vi "counter_control_multitap.vi"(0 "Downtime for pulse active":u32=20, 1 "Duration Pulse active":u32=10, 2 "Signal-high duration":u32=20, 3 "Signal-high lead-up":u32=10) -> ()   [LabVIEW 2015]
panel:
  out "Num Pulse errors":T1
  out "Configuration Error messages":T1
  # "Output"
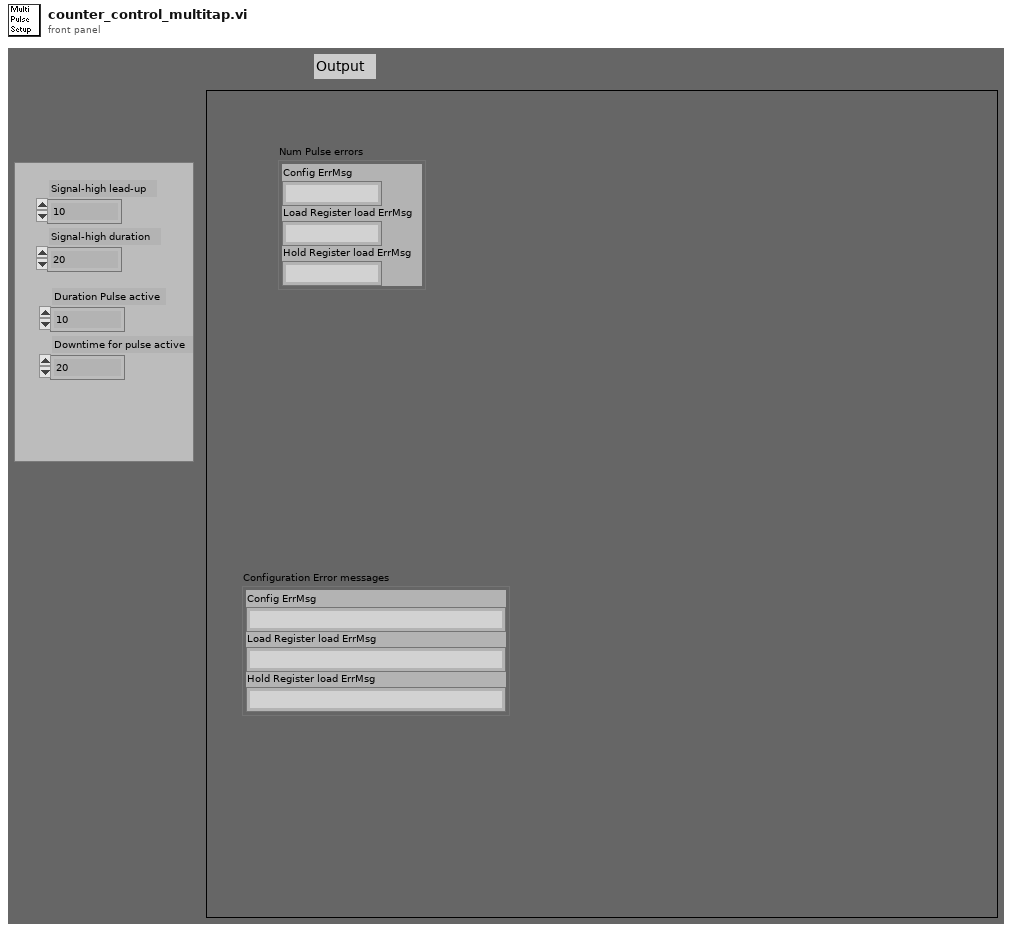
[diagram p1: front panel]
types:
  T1 = cluster{"Config ErrMsg":string, "Load Register load ErrMsg":string, "Hold Register load ErrMsg":string}
  T2 = cluster{"CounterNum":u32, "GateControl":u32, "CountSource Freq":u32, "OutputControl (LOW)":u32, "Signal-high lead-up":u32, "Signal-high duration":u32}
  T3 = cluster{"CounterNum":u32, "GateControl":u32, "CountSource Freq":u32, "OutputControl (LOW)":u32, "Duration Pulse active":u32, "Downtime for pulse active":u32}
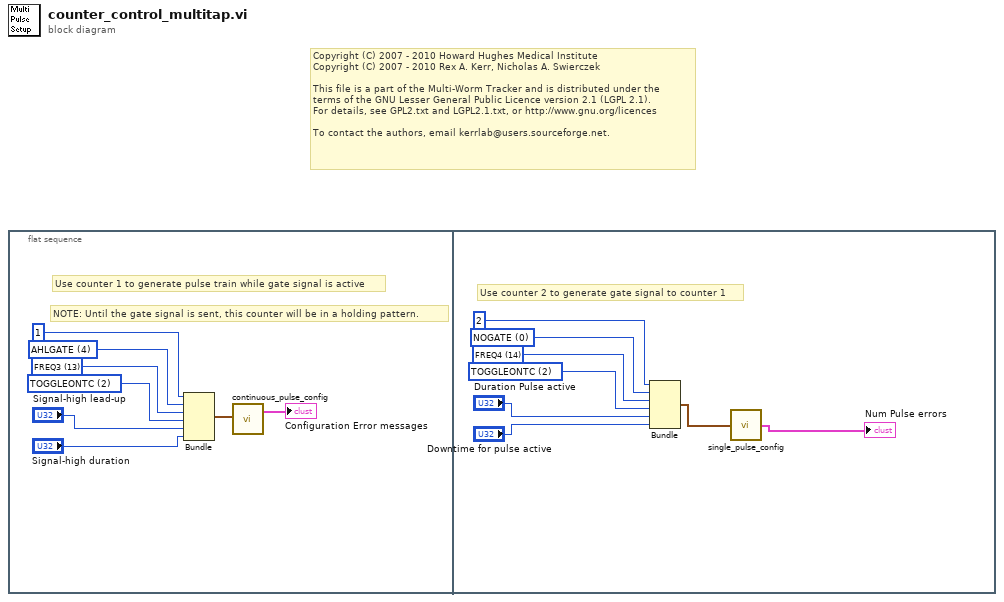
[diagram p0: block diagram]
diagram:
  # "Copyright (C) 2007 - 2010 Howard Hughes Medical Institute\nCopyright (C) 2007 - 2010 Rex A. Kerr, Nicholas A. Swierczek\n \nThis file is a part of the Multi-Worm Tracker and is distributed under the\nterms of the GNU Lesser General Public Licence version 2.1 (LGPL 2.1).\nFor details, see GPL2.txt and LGPL2.1.txt, or http://www.gnu.org/licences\n \nTo contact the authors, email kerrlab@users.sourceforge.net."
  n1 = flat-sequence {
    frame #0 {
      w5 = u32 2 items=["ALWAYSLOW", "HIGHPULSEONTC", "TOGGLEONTC", "DISCONNECTED", "LOWPULSEONTC"] ("OutputControl (LOW)")
      w6 = u32 13 items=["TCPREVCTR", "CTRINPUT1", "CTRINPUT2", "CTRINPUT3", "CTRINPUT4", "CTRINPUT5", "GATE1", "GATE2", "GATE3", "GATE4", "GATE5", "FREQ1", "FREQ2", "FREQ3", "FREQ4", "FREQ5", "CTRINPUT6", "CTRINPUT7", "CTRINPUT8", "CTRINPUT9", "CTRINPUT10", "GATE6", "GATE7", "GATE8", "GATE9", "GATE10", "FREQ6", "FREQ7", "FREQ8", "FREQ9", "FREQ10", "CTRINPUT11", "CTRINPUT12", "CTRINPUT13", "CTRINPUT14", "CTRINPUT15", "GATE11", "GATE12", "GATE13", "GATE14", "GATE15", "FREQ11", "FREQ12", "FREQ13", "FREQ14", "FREQ15", "CTRINPUT16", "CTRINPUT17", "CTRINPUT18", "CTRINPUT19", "CTRINPUT20", "GATE16", "GATE17", "GATE18", "GATE19", "GATE20", "FREQ16", "FREQ17", "FREQ18", "FREQ19", "FREQ20"] ("CountSource Freq")
      w7 = u32 4 items=["NOGATE", "AHLTCPREVCTR", "AHLNEXTGATE", "AHLPREVGATE", "AHLGATE", "ALLGATE", "AHEGATE", "ALEGATE"] ("GateControl")
      # "Use counter 1 to generate pulse train while gate signal is active"
      # "NOTE: Until the gate signal is sent, this counter will be in a holding pattern."
      n2 = Bundle("CounterNum"=u32 1, "GateControl"=w7, "CountSource Freq"=w6, "OutputControl (LOW)"=w5, "Signal-high lead-up"="Signal-high lead-up", "Signal-high duration"="Signal-high duration") -> (w1:T2)  [unwired: 1 in]
      n3 = call "continuous_pulse_config.vi"("output cluster"=w1) -> ("Error output"=→"Configuration Error messages":T1)
    }
    frame #1 {
      w16 = u32 2 items=["ALWAYSLOW", "HIGHPULSEONTC", "TOGGLEONTC", "DISCONNECTED", "LOWPULSEONTC"] ("OutputControl (LOW)")
      w15 = u32 14 items=["TCPREVCTR", "CTRINPUT1", "CTRINPUT2", "CTRINPUT3", "CTRINPUT4", "CTRINPUT5", "GATE1", "GATE2", "GATE3", "GATE4", "GATE5", "FREQ1", "FREQ2", "FREQ3", "FREQ4", "FREQ5", "CTRINPUT6", "CTRINPUT7", "CTRINPUT8", "CTRINPUT9", "CTRINPUT10", "GATE6", "GATE7", "GATE8", "GATE9", "GATE10", "FREQ6", "FREQ7", "FREQ8", "FREQ9", "FREQ10", "CTRINPUT11", "CTRINPUT12", "CTRINPUT13", "CTRINPUT14", "CTRINPUT15", "GATE11", "GATE12", "GATE13", "GATE14", "GATE15", "FREQ11", "FREQ12", "FREQ13", "FREQ14", "FREQ15", "CTRINPUT16", "CTRINPUT17", "CTRINPUT18", "CTRINPUT19", "CTRINPUT20", "GATE16", "GATE17", "GATE18", "GATE19", "GATE20", "FREQ16", "FREQ17", "FREQ18", "FREQ19", "FREQ20"] ("CountSource Freq")
      w14 = u32 0 items=["NOGATE", "AHLTCPREVCTR", "AHLNEXTGATE", "AHLPREVGATE", "AHLGATE", "ALLGATE", "AHEGATE", "ALEGATE"] ("GateControl")
      # "Use counter 2 to generate gate signal to counter 1"
      n4 = Bundle("CounterNum"=u32 2, "GateControl"=w14, "CountSource Freq"=w15, "OutputControl (LOW)"=w16, "Duration Pulse active"="Duration Pulse active", "Downtime for pulse active"="Downtime for pulse active") -> (w12:T3)  [unwired: 1 in]
      n5 = call "single_pulse_config.vi"("output cluster"=w12) -> ("Error output"=→"Num Pulse errors":T1)
    }
  }
